vi "Camera_Image_Utility.vi"() -> ()   [LabVIEW 2015]
uses:
  Camera Server/Camera enum/Camera enum.ctl
  Anemometry Sub Vis/File/Setup_Filetype.ctl
  Anemometry Sub Vis/Gen Trav/Trav_mode.ctl
panel:
  in  "Traverse Name":string="EnFlo_Stack"
  in  "Datum Position":sgl[](array[numeric])=[0.0, 0.0, 50.0] format="%#.2f"
  out "Message":string
  in  "Mode":T1(ring)
  in  "Duration (s)":dbl=5.0 format="%#_13g"
  in  "Averaging time (s) (from end)":dbl=1.0 format="%#_13g"
  in  "Camera":T2="Travcam"
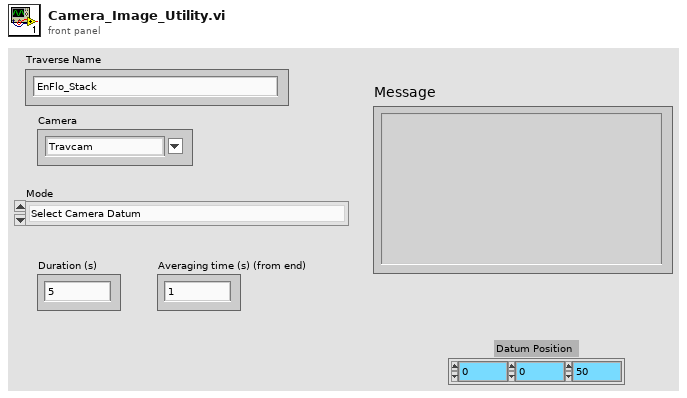
[diagram p1: front panel]
types:
  T1 = enum16{"Select Camera Datum", "Teach Datum offset from Traverse Origin"}
  T2 = typedef "Camera enum.ctl" = string
  T3 = typedef "Setup_Filetype.ctl" = enum16{"Measurement Setups", "Calibration Setups", "General", "Results File Plotter Setups", "Speed Calib Tweaks"}
  T4 = typedef "Trav_mode.ctl" = enum16{"Move traverse", "Read traverse position", "Teach Position"}
  T5 = typedef "ROI bounds.ctl" = cluster{"Xmax":i32, "Ymax":i32, "Xmin":i32, "Ymin":i32}
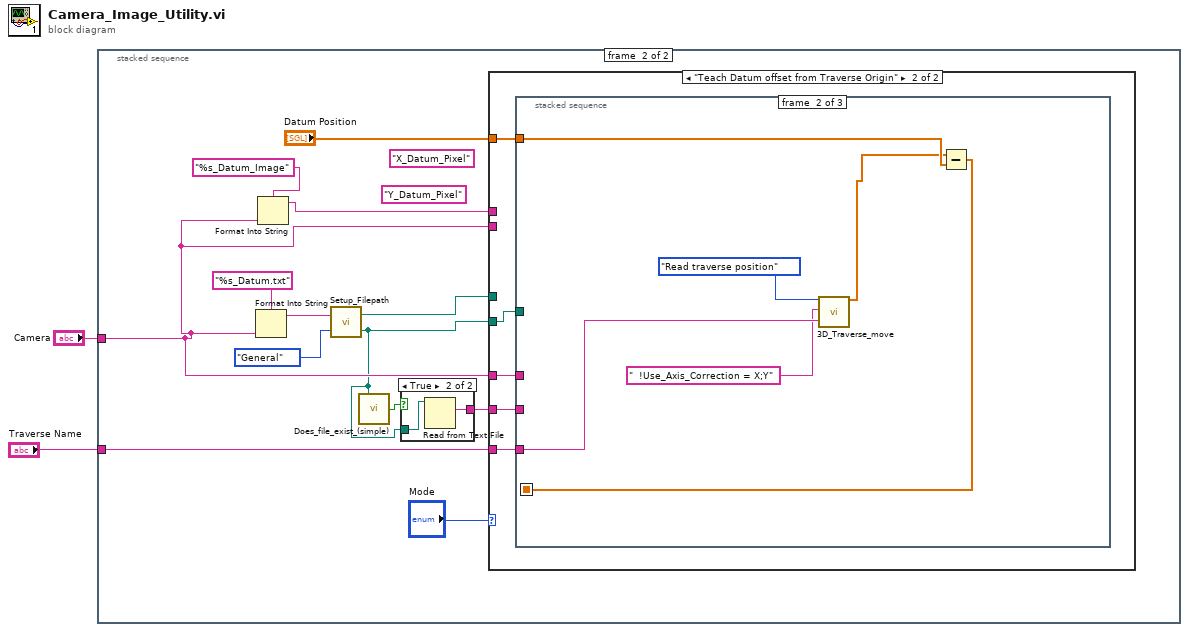
[diagram p0: block diagram]
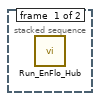
[diagram p2: hidden frame]
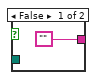
[diagram p3: hidden frame]
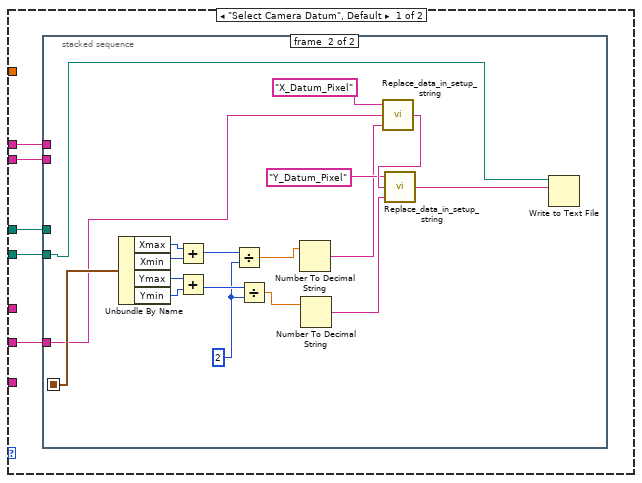
[diagram p4: hidden frame]
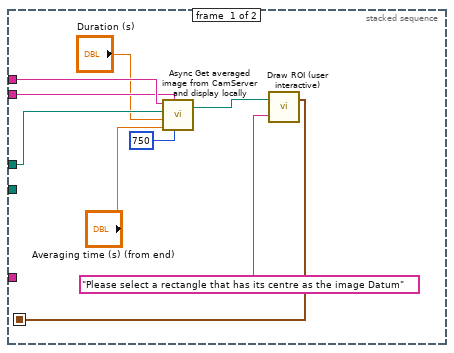
[diagram p5: hidden frame]
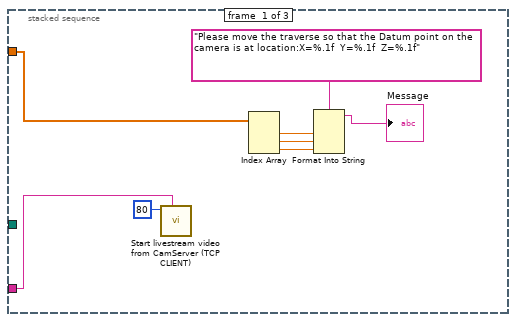
[diagram p6: hidden frame]
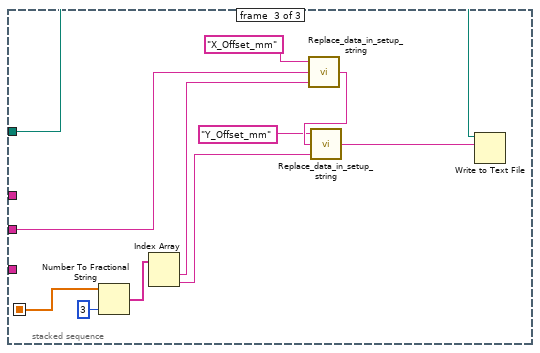
[diagram p7: hidden frame]
diagram:
  n1 = stacked-sequence {
    tunnel: "Camera" -> [_ w8]
    tunnel: "Traverse Name" -> [_ w6]
    frame #0 {
      n2 = call "Run_EnFlo_Hub.vi"() -> ()  [unwired: 8 in]
    }
    frame #1 {
      (unwired) "Y_Datum_Pixel" ("Variable name")
      (unwired) "X_Datum_Pixel" ("Variable name")
      n3 = Format Into String(format string="%s_Datum.txt", w8) -> (resulting string=w15:string)  [unwired: 2 in, 1 out]
      n4 = Format Into String(format string="%s_Datum_Image", w8) -> (resulting string=w10:string)  [unwired: 2 in, 1 out]
      n5 = call "Setup_Filepath.vi"("Setup File Type"=Setup_Filetype."General", "Filename in"=w15) -> ("Filename Out"=w3:path, "Directory"=w11:path)
      n6 = call "Does_file_exist_(simple).vi"("Pathname"=w3) -> ("exists?"=w5:bool)
      n7 = case shown="True" w5 {
        tunnel: ["" w18] -> w4
        tunnel: w3 -> [_ w17]
        frame False {
        }
        frame True {
          n8 = Read from Text File(file (use dialog)=w17) -> (text=w18:string)  [unwired: 3 in, 3 out]
        }
      }
      n9 = case shown="\"Teach Datum offset from Traverse Origin\"" "Mode" {
        tunnel: w11 -> [w23 _]
        tunnel: w10 -> [w22 _]
        tunnel: w3 -> [w21 w52]
        tunnel: w8 -> [w20 _]
        tunnel: w8 -> [_ w55]
        tunnel: "Datum Position" -> [_ w54]
        tunnel: w6 -> [_ w53]
        tunnel: w4 -> [w19 w51]
        frame "Select Camera Datum", Default {
          n10 = stacked-sequence {
            seq-local: [w25 _] -> [_ w50]
            tunnel: w23 -> [w32 _]
            tunnel: w22 -> [w31 _]
            tunnel: w20 -> [w30 _]
            tunnel: w21 -> [_ w33]
            tunnel: w19 -> [_ w34]
            frame #0 {
              n11 = call "Async Get averaged image from CamServer and display locally.vi"("Quality"=u32 750, "Camera"=w30, "Averaging time (s) (from end)"="Averaging time (s) (from end)", "Duration (s)"="Duration (s)", "Image directory path"=w32, "Image name"=w31) -> ("Image file path"=w26:path)  [unwired: 1 out]
              n12 = call "Draw ROI (user interactive).vi"("Dialog title message"="Please select a rectangle that has its centre as the image Datum", "Image file path"=w26) -> ("ROI to crop (pixels)"=w25:T5)  [unwired: 1 out]
            }
            frame #1 {
              w43 = 2 ("y")
              n13 = Unbundle By Name(w50) -> ("Xmax"=w48:i32, "Xmin"=w49:i32, "Ymax"=w47:i32, "Ymin"=w46:i32)
              n14 = Add(x=w48, y=w49) -> (x+y=w45:i32)
              n15 = Add(x=w47, y=w46) -> (x+y=w44:i32)
              n16 = Divide(x=w45, y=w43) -> (x/y=w38:dbl)
              n17 = Divide(x=w44, y=w43) -> (x/y=w37:dbl)
              n18 = Number To Decimal String(number=w38) -> (decimal integer string=w36:string)  [unwired: 1 in]
              n19 = Number To Decimal String(number=w37) -> (decimal integer string=w35:string)  [unwired: 1 in]
              n20 = call "Replace_data_in_setup_string.vi"("New data string"=w36, "Input string"=w34, "Variable name"="X_Datum_Pixel") -> ("Appended string"=w41:string)
              n21 = call "Replace_data_in_setup_string.vi"("New data string"=w35, "Input string"=w41, "Variable name"="Y_Datum_Pixel") -> ("Appended string"=w39:string)
              n22 = Write to Text File(file (use dialog)=w33, text=w39) -> ()  [unwired: 2 in, 3 out]
            }
          }
        }
        frame "Teach Datum offset from Traverse Origin" {
          n23 = stacked-sequence {
            seq-local: [_ w66 _] -> [_ _ w79]
            tunnel: w55 -> [w63 _ _]
            tunnel: w54 -> [w61 w65 _]
            tunnel: w53 -> [_ w68 _]
            tunnel: w52 -> [_ _ w70]
            tunnel: w51 -> [_ _ w71]
            frame #0 {
              n24 = call "Start livestream video from CamServer (TCP CLIENT).vi"("Camera"=w63, "TCP/IP port"=u16 80) -> ()  [unwired: 4 in, 1 out]
              n25 = Index Array(array=w61) -> (element #1=w60:sgl, element #2=w59:sgl, element #3=w58:sgl)  [unwired: 3 in]
              n26 = Format Into String(format string="Please move the traverse so that the Datum point on the camera is at location:X=%.1f  Y=%.1f  Z=%.1f", w60, w59, w58) -> (resulting string=→"Message":string)  [unwired: 2 in, 1 out]
            }
            frame #1 {
              n27 = call "3D_Traverse_move.vi"("Mode"=Trav_mode."Read traverse position", "Extra command String"="  !Use_Axis_Correction = X;Y", "Traverse name"=w68) -> ("Trav Position achieved"=w64:sgl[])  [unwired: 14 in, 2 out]
              n28 = Subtract(x=w64, y=w65) -> (x-y=w66:sgl[])
            }
            frame #2 {
              n29 = Number To Fractional String(number=w79, precision (6)=i16 3) -> (F-format string=w78:string[])  [unwired: 2 in]
              n30 = Index Array(array=w78) -> (element #1=w76:string, element #2=w73:string)  [unwired: 2 in]
              n31 = call "Replace_data_in_setup_string.vi"("New data string"=w76, "Input string"=w71, "Variable name"="X_Offset_mm") -> ("Appended string"=w75:string)
              n32 = call "Replace_data_in_setup_string.vi"("New data string"=w73, "Input string"=w75, "Variable name"="Y_Offset_mm") -> ("Appended string"=w72:string)
              n33 = Write to Text File(file (use dialog)=w70, text=w72) -> ()  [unwired: 2 in, 3 out]
            }
          }
        }
      }
    }
  }
